vi "Checkers Piece Drawer.vi"() -> ()   [LabVIEW 2016]
panel:
  out "new picture":picture
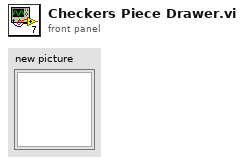
[diagram p1: front panel]
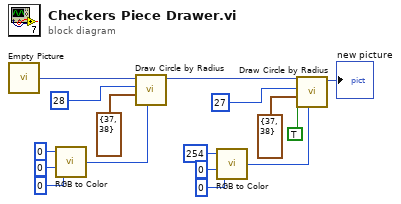
[diagram p0: block diagram]
diagram:
  n1 = call "Empty Picture"() -> ("empty picture"=w13:picture)
  n2 = call <vilib>:"RGB to Color.vi"("B"=u8 0, "G"=u8 0, "R"=u8 0) -> ("Color"=w16:u32)
  n3 = call <vilib>:"Draw Circle by Radius.vi"("color(black)"=w16, "pixel center"=cluster{"horizontal":i16, "vertical":i16} {"horizontal"=37, "vertical"=38}, "radius"=i16 28, "picture"=w13) -> ("new picture"=w3:picture)  [unwired: 7 in]
  n4 = call <vilib>:"RGB to Color.vi"("B"=u8 0, "G"=u8 0, "R"=u8 254) -> ("Color"=w4:u32)
  n5 = call <vilib>:"Draw Circle by Radius.vi"("color(black)"=w4, "fill?(F)"=TRUE, "pixel center"=cluster{"horizontal":i16, "vertical":i16} {"horizontal"=37, "vertical"=38}, "radius"=i16 27, "picture"=w3) -> ("new picture"=→"new picture":picture)  [unwired: 6 in]
